vi "Send event message.vi"(9 "Incident":refnum<class "Incident.lvclass">, 11 "RT Queues":T1) -> (3 "RT Queues out":T1)   [LabVIEW 2018]
uses:
  Type Defs/Queues cluster.ctl
  Chris VIs/Message Scheduler/message scheduler.lvclass
  Chris VIs/Incident logger/Incidents/Incident.lvclass
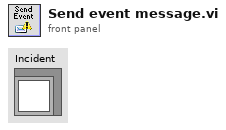
[diagram p1: front panel]
types:
  T1 = typedef "Queues cluster.ctl" = cluster{"RT Message":refnum<queue>, "RT Comms":refnum<queue>, "RT Data":refnum<queue>, "RT FIFO":refnum<queue>, "message scheduler":refnum<class "message scheduler.lvclass">}
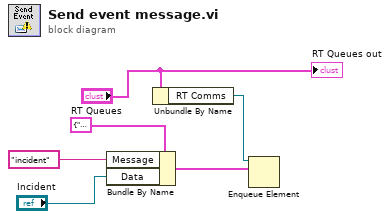
[diagram p0: block diagram]
diagram:
  n1 = Bundle By Name(cluster=cluster{"Message":string, "Data":variant} {"Message"="", "Data"=variant} ("element"), "Message"="incident", "Data"="Incident") -> (w5:cluster{"Message":string, "Data":variant})
  n2 = Unbundle By Name("RT Queues") -> ("RT Comms"=w3:refnum<queue>)
  n3 = Enqueue Element(queue=w3, element=w5) -> ()  [unwired: 2 in, 3 out]
  "RT Queues out" <- "RT Queues"
